vi "Create DVR API for Class Method.vi"(6 "DVR API Suffix":string=" API", 8 "error in (no error)":errorcluster, 9 "Class DVR Control File Path":path=path "D:/GitHub/LabVIEW/SLL/Tools/Class DVR API Generator/Temp/Class DVR Control.ctl", 10 "DVR API Directory Path":path=path "D:/GitHub/LabVIEW/SLL/Tools/Class DVR API Generator/Example/APIs", 11 "Class Method Path":path=path "D:/GitHub/LabVIEW/SLL/Tools/Class DVR API Generator/Example/Methods/Sample Class Method.vi") -> (0 "error out":errorcluster)   [LabVIEW 2016, in "SLL Class DVR API Generator.lvlib"]
uses:
  SLL Class DVR API Generator.lvlib
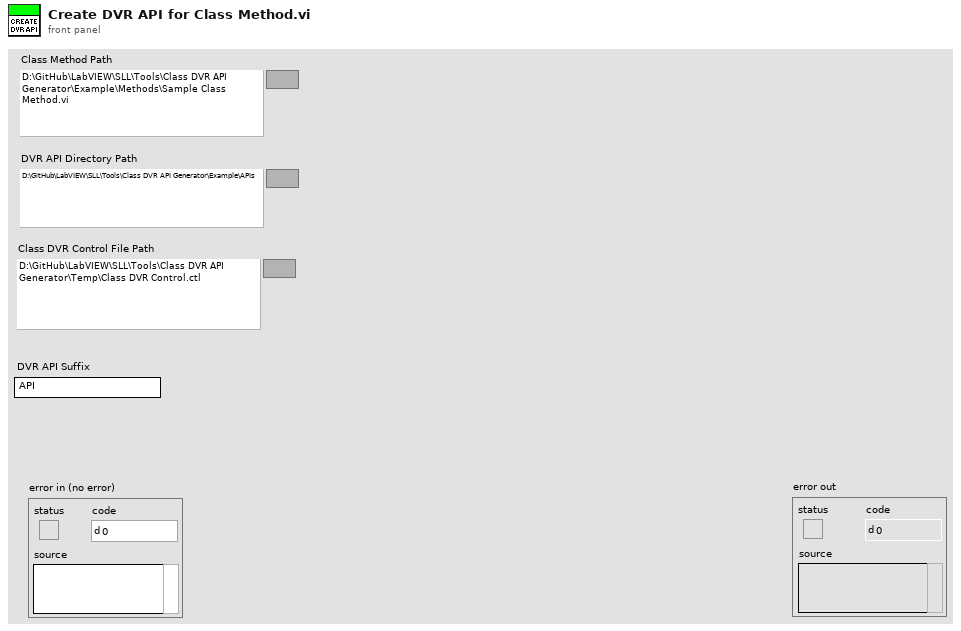
[diagram p1: front panel]
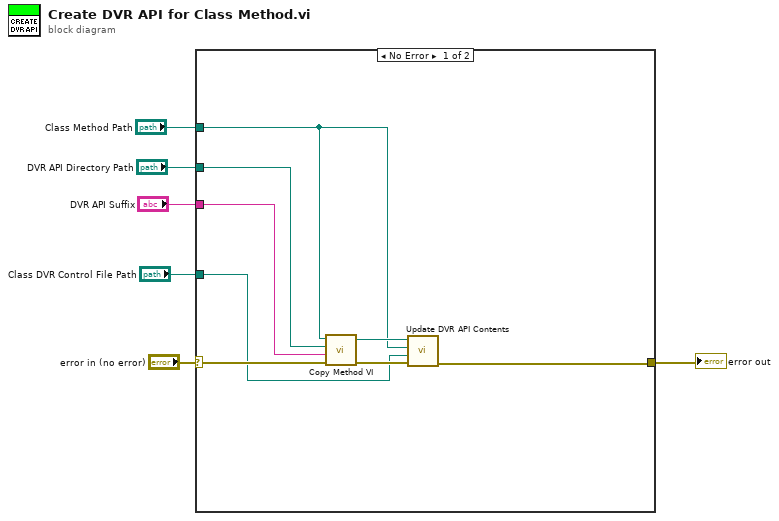
[diagram p0: block diagram]
diagram:
  n1 = case shown="No Error" "error in (no error)" {
    selector: "error in (no error)" -> [w12 w15]
    tunnel: "Class Method Path" -> [w9 _]
    tunnel: "DVR API Directory Path" -> [w14 _]
    tunnel: "DVR API Suffix" -> [w13 _]
    tunnel: [w8 w15] -> w2
    tunnel: "Class DVR Control File Path" -> [w7 _]
    frame No Error {
      n2 = call "Copy Method VI.vi"("error in (no error)"=w12, "DVR API Suffix"=w13, "DVR API Directory Path"=w14, "Class Method Path"=w9) -> ("error out"=w11:errorcluster, "DVR Method Path Out"=w10:path)  [unwired: 6 in]
      n3 = call "Update DVR API Contents.vi"("error in (no error)"=w11, "Class DVR Control File Path"=w7, "Method Path"=w9, "DVR API Path"=w10) -> ("error out"=w8:errorcluster)  [unwired: 7 in]
    }
    frame Error {
    }
  }
  "error out" <- w2
